vi "Load Settings Section.vi"(8 "Error in":errorcluster caption="Error in (no error)", 10 "Section Name":string, 11 "JSON Settings Path":path) -> (0 "Error out":errorcluster, 1 "Found":bool, 3 "JSON Object":string)   [LabVIEW 2023, in "VIDoc Settings.lvclass"]
uses:
  VIDoc Settings.lvclass
  <vilib>/JDP Science/JSONtext/Next JSON Value.vi
  <vilib>/JDP Science/JSONtext/String Subset.vi
  <vilib>/JDP Science/JSONtext/Parsing/Advance past next JSON Value (inlined COPY).vi
  <vilib>/JDP Science/JSONtext/Parsing/Advance past whitespace.vi
  <vilib>/JDP Science/JSONtext/Parsing/Advance past String.vi
  <vilib>/JDP Science/JSONtext/Parsing/Advance past Number.vi
  <vilib>/JDP Science/JSONtext/Parsing/Advance past Line Ending.vi
  <vilib>/JDP Science/JSONtext/Parsing/Parse Full Path or Item Name.vi
  <vilib>/JDP Science/JSONtext/Parsing/Advance past Array.vi
  <vilib>/JDP Science/JSONtext/Parsing/Advance past Object.vi
  <vilib>/JDP Science/JSONtext/support/Error Cluster From Code.vi
  <vilib>/JDP Science/JSONtext/Offset/Find Item Locations by Path.vi
  <vilib>/JDP Science/JSONtext/JSONtext.lvlib
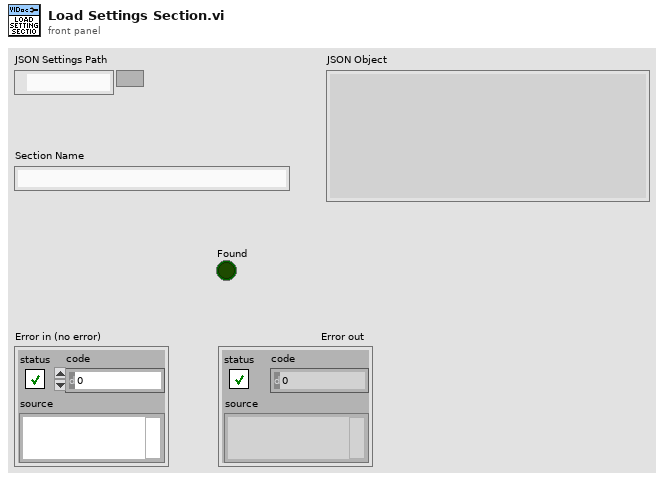
[diagram p1: front panel]
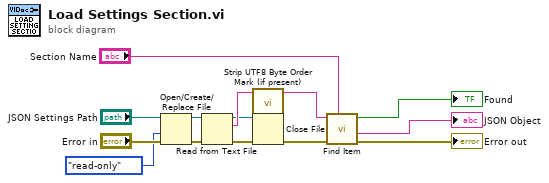
[diagram p0: block diagram]
diagram:
  n1 = Open/Create/Replace File(file path (use dialog)="JSON Settings Path", error in="Error in", access (0:read/write)=enum16{"read/write", "read-only", "write-only"}."read-only") -> (refnum out=w10:refnum<file>, error out=w11:errorcluster)  [unwired: 3 in, 1 out]
  n2 = Read from Text File(file (use dialog)=w10, error in=w11) -> (refnum out=w8:refnum<file>, text=w9:string, error out=w7:errorcluster)  [unwired: 2 in, 1 out]
  n3 = call <vilib>:"Strip UTF8 Byte Order Mark (if present).vi"("Text in"=w9) -> ("Possible Byte Order Mark Stripped"=w5:string)  [unwired: 9 in, 1 out]
  n4 = Close File(refnum=w8, error in=w7) -> (error out=w6:errorcluster)  [unwired: 1 out]
  n5 = call <vilib>:"Find Item.vi"("$Path or Item Name"="Section Name", "error in (no error)"=w6, "JSON"=w5) -> ("error out"=→"Error out":errorcluster, "<JSON>"=→"JSON Object":string, "Found"=→"Found":bool)  [unwired: 5 in, 1 out]
